vi "GetType.vi"(8 "error in (no error)":errorcluster, 11 "MoveAfterReference Msg":refnum<class "MoveAfterReference Msg.lvclass">) -> (0 "error out":errorcluster, 2 "Data Sample":variant, 3 "MoveAfterReference Msg":refnum<class "MoveAfterReference Msg.lvclass">)   [LabVIEW 2015, in "CS++Motor.lvlib" / "MoveAfterReference Msg.lvclass"]
uses:
  MoveAfterReference Msg.lvclass
  MoveAfterReference Msg.lvclass/MoveAfterReference Msg.ctl
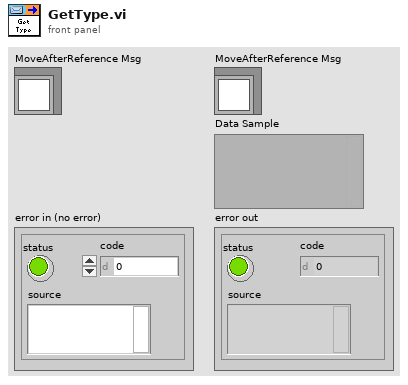
[diagram p1: front panel]
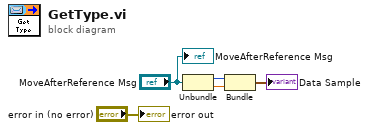
[diagram p0: block diagram]
diagram:
  n1 = Unbundle("MoveAfterReference Msg") -> (w2:u8, w1:dbl)
  n2 = Bundle("AxisNumber"=w2, "Position"=w1) -> (→"Data Sample":cluster{"AxisNumber":u8, "Position":dbl})  [unwired: 1 in]
  "error out" <- "error in (no error)"
  "MoveAfterReference Msg" <- "MoveAfterReference Msg"
